vi "getImage.vi"(8 "error in (no error)":errorcluster, 10 "stop":bool, 11 "ICCameraAcquisitor in":refnum<class "ICCameraAcquisitor.lvclass">) -> (0 "error out":errorcluster, 2 "Array":path[](array[path]), 3 "ICCameraAcquisitor out":refnum<class "ICCameraAcquisitor.lvclass">)   [LabVIEW 2011, in "Hardware.lvlib" / "Channels.lvlib" / "ICCameraAcquisitor.lvclass"]
uses:
  ICCameraAcquisitor.lvclass
  ICCameraAcquisitor.lvclass/ICCameraAcquisitor.ctl
  Tools/Filing/FileSystem/FileSystem.lvclass
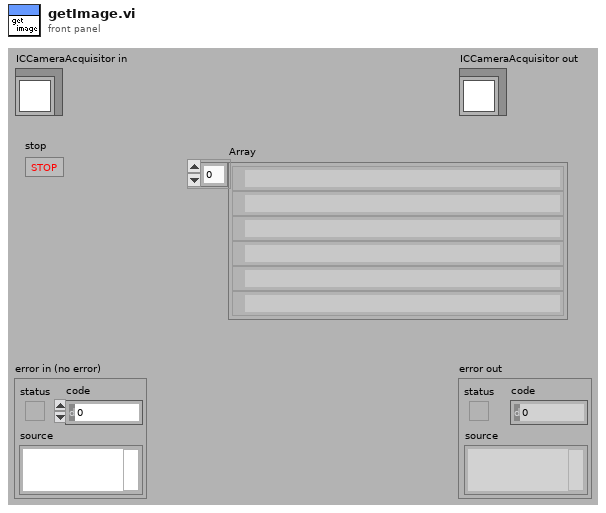
[diagram p1: front panel]
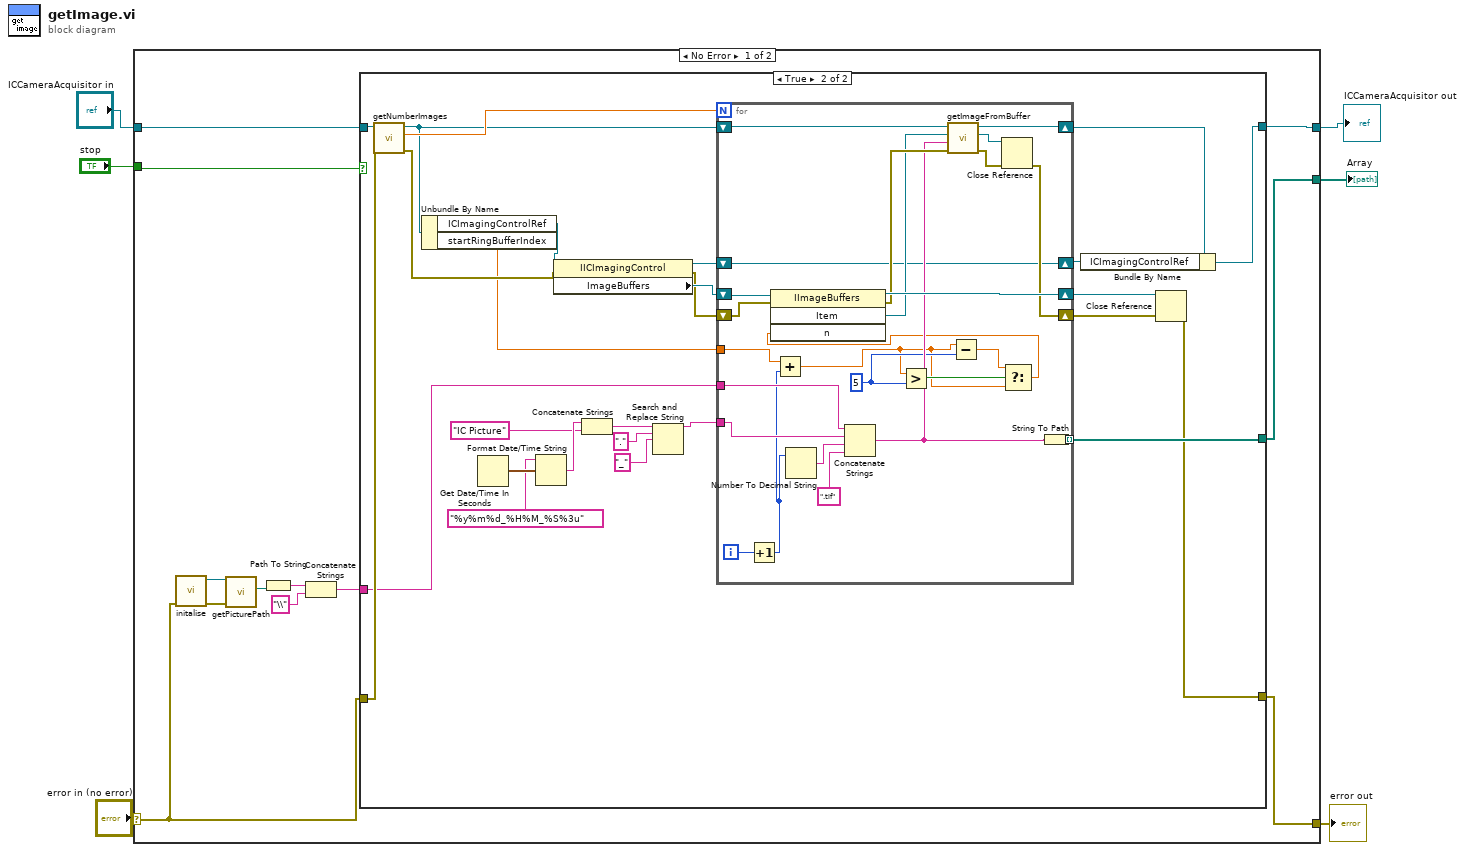
[diagram p0: block diagram]
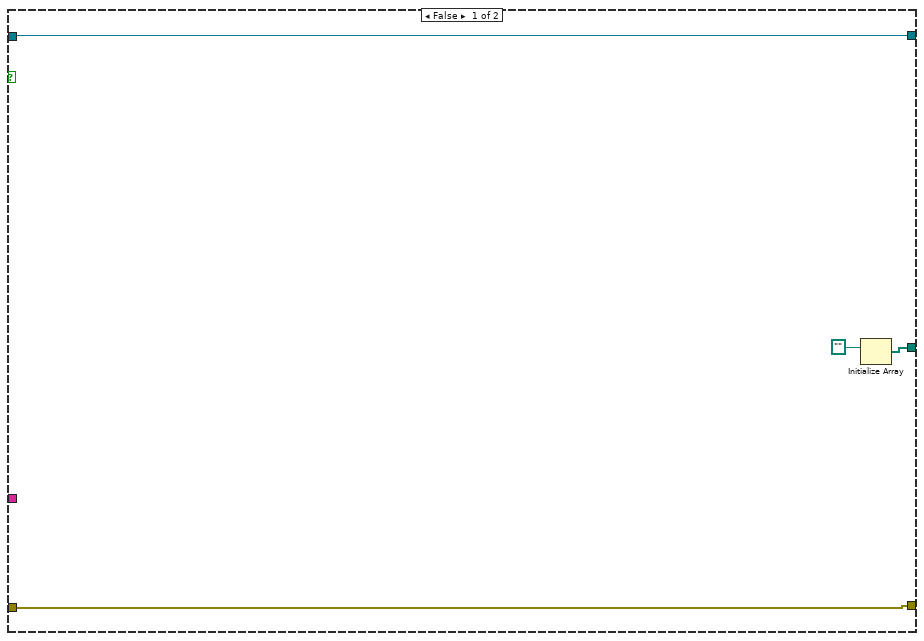
[diagram p2: hidden frame]
diagram:
  n1 = case shown="No Error" "error in (no error)" {
    selector: "error in (no error)" -> [w8 w74]
    tunnel: "ICCameraAcquisitor in" -> [w17 w75]
    tunnel: "stop" -> [w18 _]
    tunnel: [w15 w74] -> w3
    tunnel: [w16 w75] -> w2
    tunnel: [w14 _] -> w1
    frame No Error {
      n2 = call "initalise.vi"("error in (no error)"=w8) -> ("error out"=w12:errorcluster, "FileSystem out"=w13:refnum<class "FileSystem.lvclass">)  [unwired: 9 in]
      n3 = call "getPicturePath.vi"("error in (no error)"=w12, "FileSystem in"=w13) -> ("PicturePath"=w11:path)  [unwired: 7 in, 2 out]
      n4 = Path To String(path=w11) -> (string=w10:string)
      n5 = Concatenate Strings(w10, "\\") -> (w7:string)
      n6 = case shown="True" w18 {
        tunnel: w17 -> [w20 w48]
        tunnel: w8 -> [w19 w47]
        tunnel: [w20 w25] -> w16
        tunnel: [w19 w33] -> w15
        tunnel: [w21 w36] -> w14
        tunnel: w7 -> [_ w23]
        frame False {
          n7 = Initialize Array(path "") -> (w21:path[])  [unwired: 1 in]
        }
        frame True {
          n8 = call-dynamic "getNumberImages.vi"("error in (no error)"=w47, "CameraAcquisitor.lvclass in"=w48) -> ("error out"=w30:errorcluster, "Number of Images"=w46:dbl, "CameraAcquisitor.lvclass out"=w45:refnum<class "ICCameraAcquisitor.lvclass">)  [unwired: 7 in]
          n9 = Unbundle By Name(w45) -> ("ICImagingControlRef"=w32:refnum<k7>, "startRingBufferIndex"=w24:dbl)
          n10 = Get Date/Time In Seconds() -> (seconds since 1Jan1904=w39:timestamp)
          n11 = Format Date/Time String(time format string (%c)="%y%m%d_%H%M_%S%3u", seconds (now)=w39) -> (date/time string=w41:string)  [unwired: 1 in]
          n12 = property class="IICImagingControl"(reference=w32, error in=w30) -> (reference out=w28:refnum<k7>, error out=w29:errorcluster, "ImageBuffers"=w31:refnum<k7>)
          n13 = Concatenate Strings(w41, "IC Picture") -> (w42:string)
          n14 = Search and Replace String(input string=w42, search string=".", replace string="_") -> (result string=w37:string)  [unwired: 5 in, 3 out]
          n15 = for {
            N: w46 -> [_]
            shift-right: [w58] -> w35
            shift-left: w29 -> [w72]
            shift-right: [w65] -> w26
            shift-left: w45 -> [w66]
            shift-right: [w71] -> w34
            shift-left: w31 -> [w73]
            tunnel: w37 -> [w68]
            tunnel: w23 -> [w67]
            tunnel: [w61] -> w36 mode=indexing
            shift-right: [w57] -> w27
            shift-left: w28 -> [w57]
            tunnel: w24 -> [w53]
            i -> [w51]
            w56 = 5
            n16 = Increment(x=w51) -> (x+1=w49:i32)
            n17 = Add(x=w53, y=w49) -> (x+y=w52:dbl)
            n18 = Number To Decimal String(number=w49) -> (decimal integer string=w70:string)  [unwired: 1 in]
            n19 = Concatenate Strings(w67, w68, w70, ".tif") -> (w62:string)
            n20 = Greater?(x=w52, y=w56) -> (0:w54:bool)
            n21 = Subtract(x=w52, y=w56) -> (x-y=w55:dbl)
            n22 = Select(t=w55, s=w54, f=w52) -> (s? t:f=w50:dbl)
            n23 = invoke class="IImageBuffers" method="Item"(reference=w73, error in=w72, "n"=w50) -> (reference out=w71:refnum<k7>, error out=w64:errorcluster, "Item"=w63:refnum<k7>)  [unwired: 1 in, 1 out]
            n24 = call "getImageFromBuffer.vi"("error in (no error)"=w64, "String"=w62, "ImageBufferRef"=w63, "ICCameraAcquisitor in"=w66) -> ("error out"=w59:errorcluster, "ImageBufferRef out"=w60:refnum<k7>, "ICCameraAcquisitor out"=w65:refnum<class "ICCameraAcquisitor.lvclass">)  [unwired: 5 in]
            n25 = Close Reference(reference=w60, error in (no error)=w59) -> (error out=w58:errorcluster)
            n26 = String To Path(string=w62) -> (path=w61:path)
          }
          n27 = Bundle By Name(cluster=w26, "ICImagingControlRef"=w27) -> (w25:refnum<class "ICCameraAcquisitor.lvclass">)
          n28 = Close Reference(reference=w34, error in (no error)=w35) -> (error out=w33:errorcluster)
        }
      }
    }
    frame Error {
    }
  }
  "error out" <- w3
  "ICCameraAcquisitor out" <- w2
  "Array" <- w1
